vi "ReportElementList.vi"(1 "Destination":T1={"Subsystem Id"=90, "Node Id"=1, "Component Id"=1}, 2 "Source":T1={"Subsystem Id"=3, "Node Id"=1, "Component Id"=1}) -> (0 "Encoded JAUS Message":string)   [LabVIEW 2009]
uses:
  Support Files/Address.ctl
panel:
  in  "ElementsList":u16[](array[numeric])=[1, 2, 3, 4]
  out "appended array":u8[](array[numeric])
  in  "Command Code":string="D\u001b"
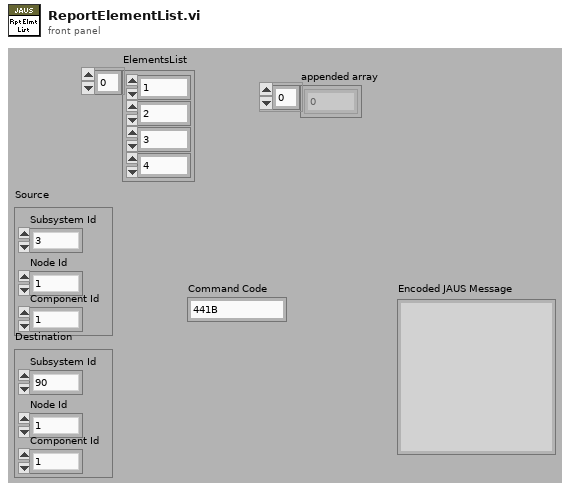
[diagram p1: front panel]
types:
  T1 = typedef "Address.ctl" = cluster{"Subsystem Id":u16, "Node Id":u8, "Component Id":u8}
  T2 = cluster{"unsigned byte array[0]":u8, "unsigned byte array[1]":u8}
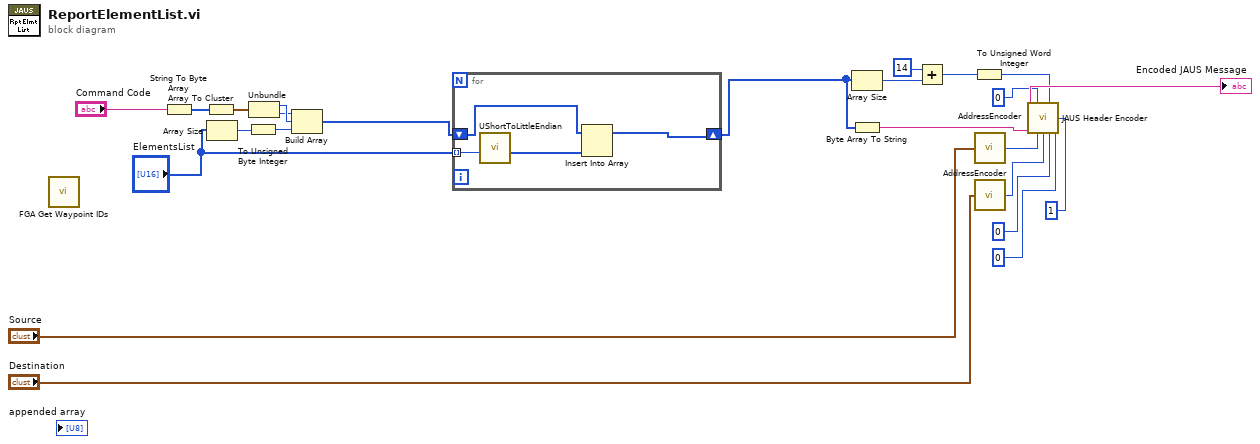
[diagram p0: block diagram]
diagram:
  n1 = call "FGA Get Waypoint IDs.vi"() -> ()  [unwired: 1 out]
  n2 = String To Byte Array(string="Command Code") -> (unsigned byte array=w19:u8[])
  n3 = Array To Cluster(array=w19) -> (cluster=w18:T2)
  n4 = Array Size(array="ElementsList") -> (size(s)=w15:i32)
  n5 = To Unsigned Byte Integer(number=w15) -> (unsigned 8bit integer=w14:u8)
  n6 = Unbundle(w18) -> ("unsigned byte array[0]"=w17:u8, "unsigned byte array[1]"=w16:u8)
  n7 = Build Array(w16, w17, w14) -> (w24:u8[])
  n8 = for {
    tunnel: "ElementsList" -> [w28] mode=indexing
    shift-right: [w26] -> w2
    shift-left: w24 -> [w25]
    n9 = call "UShortToLittleEndian.vi"("Number"=w28) -> ("byte array"=w27:u8[])  [unwired: 10 in]
    n10 = Insert Into Array(array=w25, new element=w27) -> (w26:u8[])  [unwired: 1 in]
  }
  n11 = Array Size(array=w2) -> (size(s)=w11:i32)
  n12 = Byte Array To String(unsigned byte array=w2) -> (string=w9:string)
  n13 = Add(x=14, y=w11) -> (x+y=w12:i32)
  n14 = To Unsigned Word Integer(number=w12) -> (unsigned 16bit integer=w13:u16)
  n15 = call "AddressEncoder.vi"("Address Cluster"="Source") -> ("Address"=w3:u32)
  n16 = call "AddressEncoder.vi"("Address Cluster"="Destination") -> ("Address"=w4:u32)
  n17 = call "JAUS Header Encoder.vi"("Message Type (0-5)"=u8 0, "Data Size (8-23)"=w13, "Priority(40-41)"=u8 1, "Payload"=w9, "Source ID (80-95)"=w3, "Destination ID (48-79)"=w4, "Data Flags (46-47)"=u8 0, "Ack/Nak (44-45)"=u8 0) -> ("Encoded JAUS Message"=→"Encoded JAUS Message":string)  [unwired: 7 in]
